vi "myRIO_Brig_RT__Case_Exp_State_initTrial.vi"(7 "input_spout":enum16{"Left", "Right"}(ring), 10 "input_dataExp":u16[](array[numeric]), 11 "input_dataCurrent":u16[](array[numeric])) -> (1 "output_state":T1=enum."ENL1_pre", 2 "output_dataExp":u16[](array[numeric]), 3 "output_dataCurrent":u16[](array[numeric]))   [LabVIEW 2014]
uses:
  myRIO_BRig_RT__Case_Exp_stateList.ctl
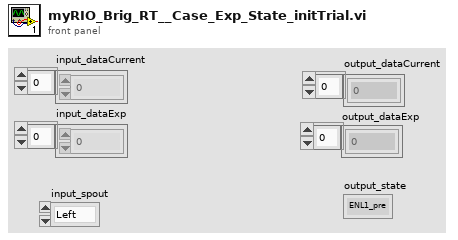
[diagram p1: front panel]
types:
  T1 = typedef "myRIO_BRig_RT__Case_Exp_stateList.ctl" = enum16{"Start1", "Start2", "Start3", "saveSettings1", "saveSettings2", "saveSettings3", "saveSettings4", "saveSettings_LC_ENL_l1", "saveSettings_LC_ENL_l2", "saveSettings_LC_Cue_l1", "saveSettings_LC_Cue_l2", "saveSettings6_LC_l1_Other", "SaveSettings6_LC_l2_Other", "setSettings_Audio", "setSettings_Laser", "initBlock_pre", "initBlock", "initBlock2", "initBlock_post", "initTrial_pre", "initTrial", "initTrial2", "initTrial3", "initTrial4", "initTrial_LC_ENL1", "initTrial_LC_Cue1", "initTrial_LC_Cue1_2", "initTrial_LC_Sel", "initTrial_post", "ENL1_pre", "ENL1", "ENL1_post", "ENL1Penalty_pre", "ENL1Penalty", "ENL2_pre", "ENL2", "ENL2Penalty_pre", "ENL2Penalty", "Cue1_pre", "Cue1", "Cue1_post", "Cue1Penalty_pre", "Cue1Penalty", "Cue2_pre", "Cue2", "Cue2Penalty_pre", "Cue2Penalty", "Selection_pre", "Selection", "Select_post", "SelectReward_pre", "SelectReward", "SelectRewardPost_pre", "SelectRewardPost", "SelectWrong_pre", "SelectWrong", "SelectWrong_post", "SelectTimeout_pre", "SelectTimeout", "SelectTimeout_post", "endTrial_pre", "endTrial1", "endTrial2", "endTrial3", "endTrial_post", "endBlock_pre", "endBlock", "endBlock_post", "endExp", "commConnect", "commUpload_pre", "commUpload_dataBlock", "commUpload_dataCurrent", "commUpload_dataExp", "commUpload_dataLC", "commUpload_dataTrial", "commUpload_post", "saveData_pre", "saveData_dataBlock", "saveData_dataCurrent", "saveData_dataExp", "saveData_dataLC", "saveData_dataTrial", "saveData_post", "empty_endBlock1", "empty_endBlock2", "empty_endTrial1", "empty_endTrial2", "empty_endTrial3", "empty_endTrial4", "empty_endTrial5", "dummyState", "dummyState_endBlock"}
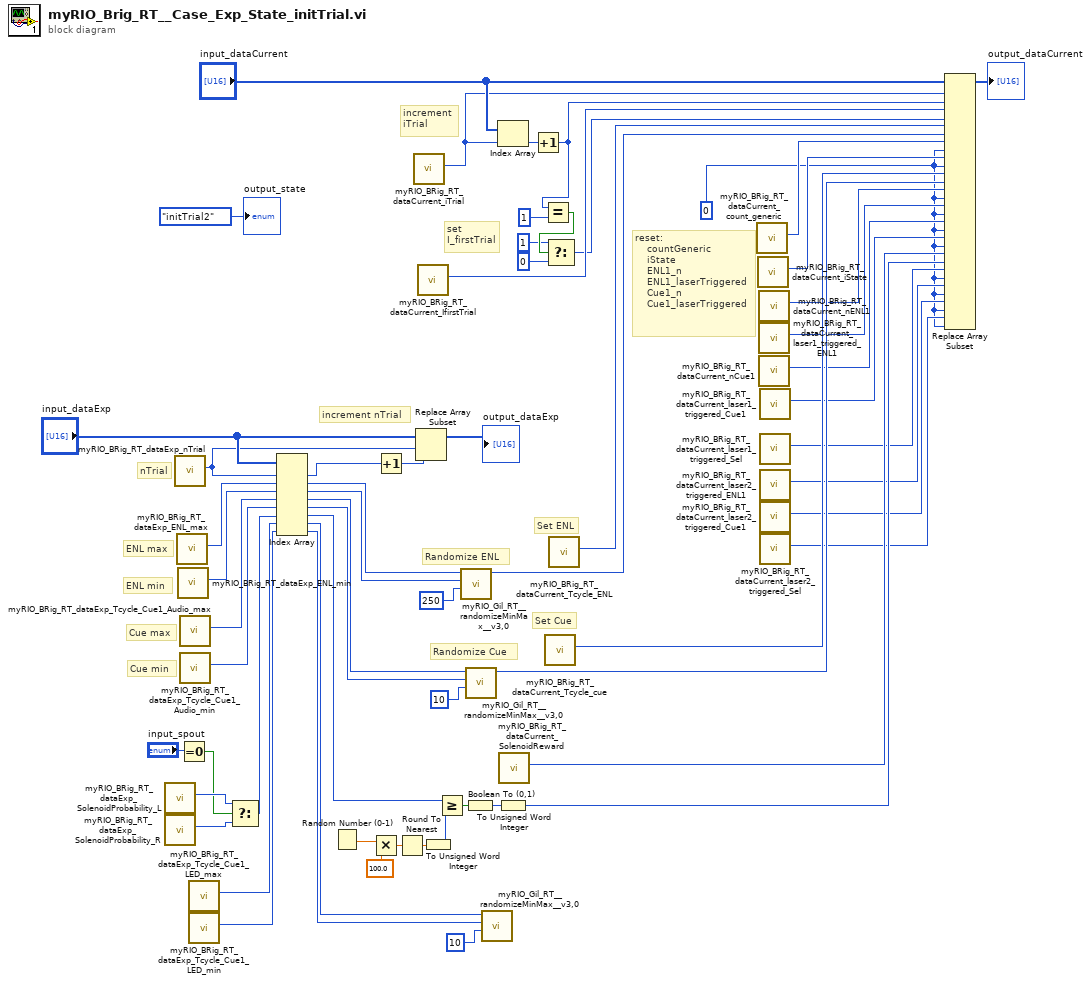
[diagram p0: block diagram]
diagram:
  w6 = u16 0 ("new element/subarray")
  # "Set Cue"
  # "Randomize Cue"
  # "Cue min"
  # "Cue max"
  # "ENL min"
  # "ENL max"
  # "nTrial"
  # "reset:\n    countGeneric\n    iState\n    ENL1_n\n    ENL1_laserTriggered\n    Cue1_n\n    Cue1_laserTriggered"
  # "increment nTrial"
  # "set\nI_firstTrial"
  # "increment\niTrial"
  # "Randomize ENL"
  # "Set ENL"
  n1 = call "myRIO_BRig_RT_dataExp_SolenoidProbability_L.vi"() -> ("output_SolenoidProbability_L"=w25:i32)  [unwired: 11 in]
  n2 = call "myRIO_BRig_RT_dataExp_SolenoidProbability_R.vi"() -> ("output_SolenoidProbability_R"=w24:i32)  [unwired: 11 in]
  n3 = call "myRIO_BRig_RT_dataExp_nTrial.vi"() -> ("output_nTrial"=w42:i32)  [unwired: 11 in]
  n4 = call "myRIO_BRig_RT_dataExp_ENL_max.vi"() -> ("output_ENL_max"=w41:i32)  [unwired: 11 in]
  n5 = call "myRIO_BRig_RT_dataExp_ENL_min.vi"() -> ("output_ENL_min"=w40:i32)  [unwired: 11 in]
  n6 = Equal To 0?(x="input_spout") -> (x = 0?=w22:bool)
  n7 = call "myRIO_BRig_RT_dataExp_Tcycle_Cue1_Audio_max.vi"() -> ("output_Tcycle_Cue1_Audio_max"=w36:i32)  [unwired: 11 in]
  n8 = call "myRIO_BRig_RT_dataExp_Tcycle_Cue1_Audio_min.vi"() -> ("output_Tcycle_Cue1_Audio_min"=w35:i32)  [unwired: 11 in]
  n9 = call "myRIO_BRig_RT_dataExp_Tcycle_Cue1_LED_max.vi"() -> ("output_Tcycle_Cue1_LED_max"=w5:i32)  [unwired: 11 in]
  n10 = call "myRIO_BRig_RT_dataExp_Tcycle_Cue1_LED_min.vi"() -> ("output_Tcycle_Cue1_LED_min"=w4:i32)  [unwired: 11 in]
  n11 = Select(t=w25, s=w22, f=w24) -> (s? t:f=w21:i32)
  n12 = Index Array(array="input_dataExp", index #1=w42, index #2=w41, index #3=w40, index #4=w36, index #5=w35, index #6=w21, index #7=w5, index #8=w4) -> (element #1=w39:u16, element #2=w38:u16, element #3=w37:u16, element #4=w33:u16, element #5=w32:u16, element #6=w15:u16, element #7=w2:u16, element #8=w1:u16)
  n13 = Random Number (0-1)() -> (number: 0 to 1=w20:dbl)
  n14 = Multiply(x=w20, y=100.0) -> (x*y=w19:dbl)
  n15 = Increment(x=w39) -> (x+1=w49:u16)
  n16 = Round To Nearest(number=w19) -> (nearest integer value=w18:dbl)
  n17 = call "myRIO_BRig_RT_dataCurrent_iTrial.vi"() -> ("output_iTrial"=w58:i32)  [unwired: 11 in]
  n18 = Replace Array Subset(array="input_dataExp", new element=w49, index=w42) -> (→"output_dataExp":u16[])
  n19 = call "myRIO_BRig_RT_dataCurrent_IfirstTrial.vi"() -> ("output_I_firstTrial"=w57:i32)  [unwired: 11 in]
  n20 = To Unsigned Word Integer(number=w18) -> (unsigned 16bit integer=w17:u16)
  n21 = Greater Or Equal?(x=w15, y=w17) -> (x >= y?=w13:bool)
  n22 = call "myRIO_Gil_RT__randomizeMinMax__v3,0.vi"("Input_Increment"=u16 250, "Input_Min"=w37, "Input_Max"=w38) -> ("Output"=w46:u16)  [unwired: 8 in]
  n23 = Boolean To (0,1)(Boolean=w13) -> (0, 1=w14:i16)
  n24 = call "myRIO_Gil_RT__randomizeMinMax__v3,0.vi"("Input_Increment"=u16 10, "Input_Min"=w32, "Input_Max"=w33) -> ("Output"=w30:u16)  [unwired: 8 in]
  n25 = call "myRIO_Gil_RT__randomizeMinMax__v3,0.vi"("Input_Increment"=u16 10, "Input_Min"=w1, "Input_Max"=w2) -> ()  [unwired: 8 in, 1 out]
  n26 = Index Array(array="input_dataCurrent", index=w58) -> (element=w59:u16)
  n27 = To Unsigned Word Integer(number=w14) -> (unsigned 16bit integer=w11:u16)
  n28 = call "myRIO_BRig_RT_dataCurrent_SolenoidReward.vi"() -> ("output_SolenoidReward"=w12:i32)  [unwired: 11 in]
  n29 = Increment(x=w59) -> (x+1=w56:u16)
  n30 = Equal?(x=w56, y=u16 1) -> (x = y?=w54:bool)
  n31 = call "myRIO_BRig_RT_dataCurrent_Tcycle_cue.vi"() -> ("output_Tcycle_cue"=w31:i32)  [unwired: 11 in]
  n32 = Select(t=u16 1, s=w54, f=u16 0) -> (s? t:f=w53:u16)
  n33 = call "myRIO_BRig_RT_dataCurrent_Tcycle_ENL.vi"() -> ("output_ENL"=w47:i32)  [unwired: 11 in]
  n34 = call "myRIO_BRig_RT_dataCurrent_count_generic.vi"() -> ("output_count_generic"=w45:i32)  [unwired: 11 in]
  n35 = call "myRIO_BRig_RT_dataCurrent_iState.vi"() -> ("output_iState"=w43:i32)  [unwired: 11 in]
  n36 = call "myRIO_BRig_RT_dataCurrent_nENL1.vi"() -> ("output_nENL1"=w29:i32)  [unwired: 11 in]
  n37 = call "myRIO_BRig_RT_dataCurrent_laser1_triggered_ENL1.vi"() -> ("output_laser1_triggered_ENL1"=w28:i32)  [unwired: 11 in]
  n38 = call "myRIO_BRig_RT_dataCurrent_nCue1.vi"() -> ("output_nCue1"=w27:i32)  [unwired: 11 in]
  n39 = call "myRIO_BRig_RT_dataCurrent_laser1_triggered_Cue1.vi"() -> ("output_laser1_triggered_Cue1"=w26:i32)  [unwired: 11 in]
  n40 = call "myRIO_BRig_RT_dataCurrent_laser1_triggered_Sel.vi"() -> ("output_laser1_triggered_Selection"=w10:i32)  [unwired: 11 in]
  n41 = call "myRIO_BRig_RT_dataCurrent_laser2_triggered_ENL1.vi"() -> ("output_laser2_triggered_ENL1"=w9:i32)  [unwired: 11 in]
  n42 = call "myRIO_BRig_RT_dataCurrent_laser2_triggered_Cue1.vi"() -> ("output_laser2_triggered_Cue1"=w8:i32)  [unwired: 11 in]
  n43 = call "myRIO_BRig_RT_dataCurrent_laser2_triggered_Sel.vi"() -> ("output_laser2_triggered_Selection"=w7:i32)  [unwired: 11 in]
  n44 = Replace Array Subset(array="input_dataCurrent", new element #1=w56, index #1=w58, new element #2=w53, index #2=w57, new element #3=w46, index #3=w47, new element #4=w6, index #4=w45, new element #5=w6, index #5=w43, new element #6=w30, index #6=w31, new element #7=w6, index #7=w29, new element #8=w6, index #8=w28, new element #9=w6, index #9=w27, new element #10=w6, index #10=w26, new element #11=w11, index #11=w12, new element #12=w6, index #12=w10, new element #13=w6, index #13=w9, new element #14=w6, index #14=w8, new element #15=w6, index #15=w7) -> (→"output_dataCurrent":u16[])
  "output_state" <- myRIO_BRig_RT__Case_Exp_stateList."initTrial2" ("Enum")
